vi "Message_Handler.vi"(7 "Action":T5, 8 "error in (no error)":errorcluster, 9 "Time_Out":i32, 11 "Message_IN":T1) -> (0 "error out":errorcluster, 3 "Message_OUT":T1)   [LabVIEW 2024, in "Camera.lvlib" / "Message_Handler.lvlib"]
uses:
  Message_Handler.lvlib
  typedeff_CommunicationModuleAction.ctl
  typedeff_Message.ctl
  typedeff_Message_Command.ctl
  typedeff_Message_Parameters.ctl
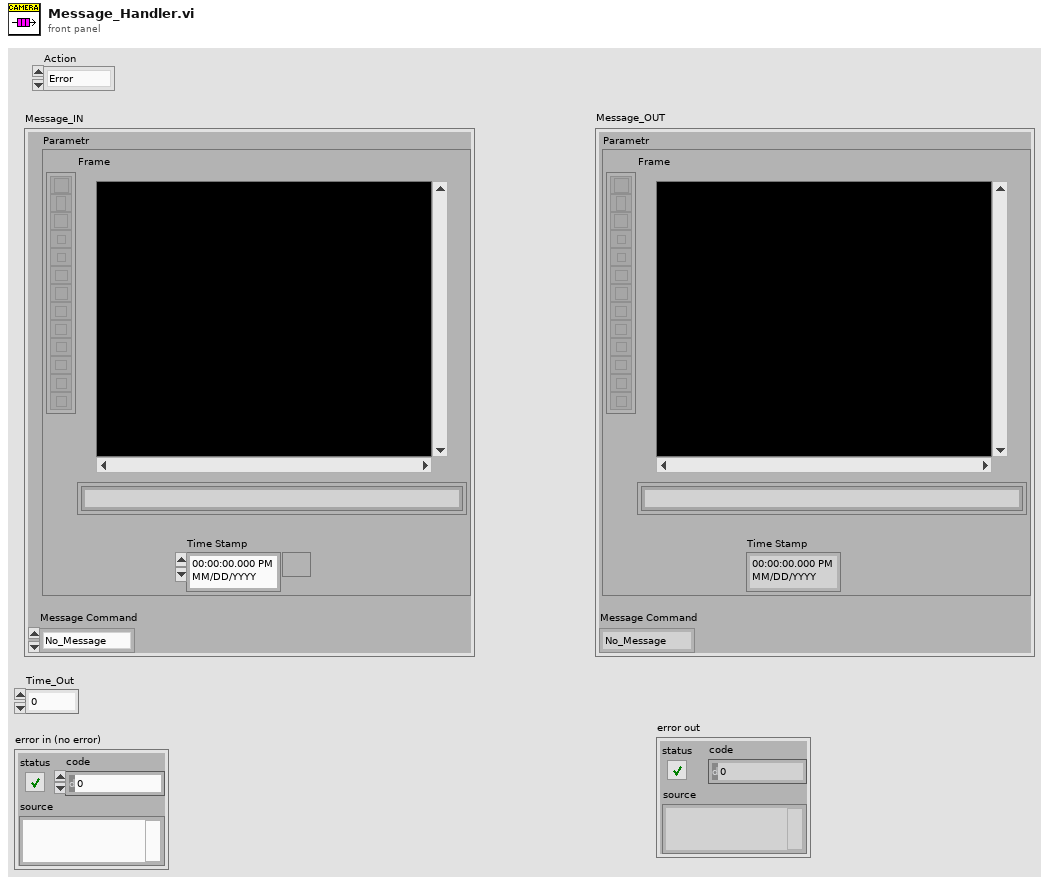
[diagram p1: front panel]
types:
  T1 = typedef "Camera.lvlib/Message_Handler.lvlib/typedeff_Message.ctl" = cluster{"Message Command":T2, "Parametr":T3}
  T2 = typedef "Camera.lvlib/Message_Handler.lvlib/typedeff_Message_Command.ctl" = enum16{"No_Message", "Send_photo"}
  T3 = typedef "Camera.lvlib/Message_Handler.lvlib/typedeff_Message_Parameters.ctl" = cluster{"Frame":T4, "Time Stamp":timestamp}
  T4 = typedef "IMAQ Image.ctl" = refnum<image>
  T5 = typedef "Camera.lvlib/Message_Handler.lvlib/typedeff_CommunicationModuleAction.ctl" = enum16{"Error", "Init", "Send Msg", "Recive Msg", "Shut Down"}
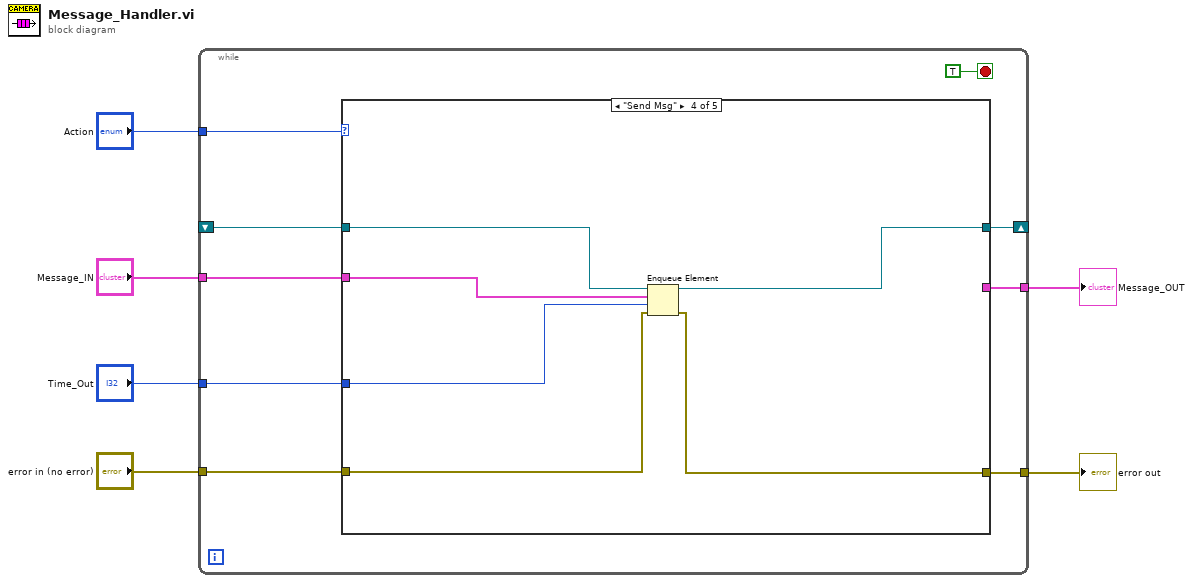
[diagram p0: block diagram]
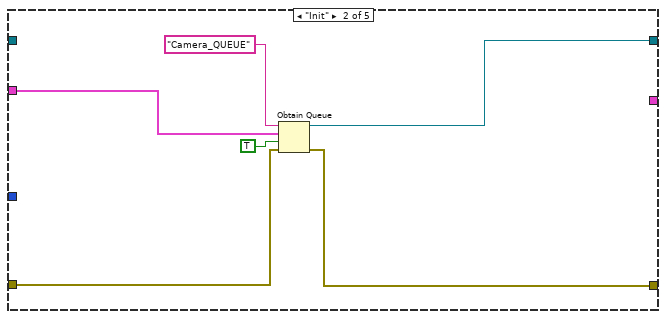
[diagram p3: hidden frame]
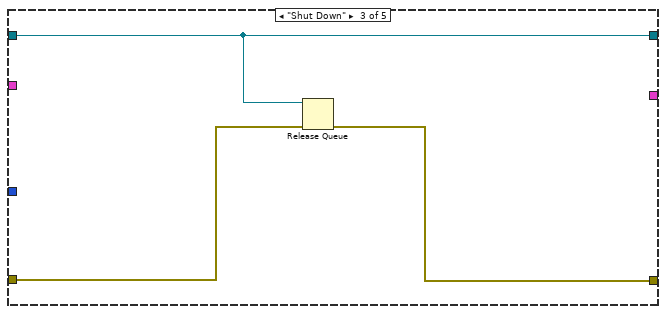
[diagram p4: hidden frame]
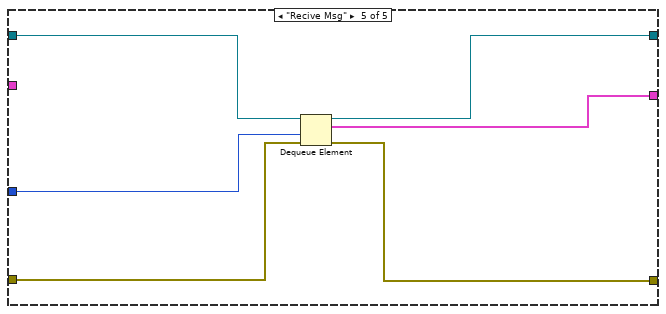
[diagram p5: hidden frame]
diagram:
  n1 = while {
    tunnel: "Action" -> [w14]
    tunnel: "error in (no error)" -> [w13]
    shift-right: [w12] -> _
    shift-left: _ -> [w11]
    tunnel: [w10] -> w4
    tunnel: "Time_Out" -> [w9]
    tunnel: [w8] -> w2
    tunnel: "Message_IN" -> [w7]
    stop <- TRUE stop-if-true
    n2 = case shown="\"Send Msg\"" w14 {
      tunnel: w13 -> [_ w21 w25 w28 w32]
      tunnel: [w16 w20 w23 w29 w35] -> w12
      tunnel: w11 -> [w16 _ w23 w31 w37]
      tunnel: [_ w19 w24 w27 w33] -> w10
      tunnel: w9 -> [_ _ _ w30 w36]
      tunnel: [_ _ _ _ w34] -> w8
      tunnel: w7 -> [_ w17 _ w26 _]
      frame "Error", Default {
      }
      frame "Init" {
        n3 = Obtain Queue(name (unnamed)="Camera_QUEUE", element data type=w17, create if not found? (T)=TRUE, error in (no error)=w21) -> (queue out=w20:refnum<queue>, error out=w19:errorcluster)  [unwired: 1 in, 1 out]
      }
      frame "Shut Down" {
        n4 = Release Queue(queue=w23, error in (no error)=w25) -> (error out=w24:errorcluster)  [unwired: 1 in, 2 out]
      }
      frame "Send Msg" {
        n5 = Enqueue Element(queue=w31, element=w26, timeout in ms (-1)=w30, error in (no error)=w28) -> (queue out=w29:refnum<queue>, error out=w27:errorcluster)  [unwired: 1 out]
      }
      frame "Recive Msg" {
        n6 = Dequeue Element(queue=w37, timeout in ms (-1)=w36, error in (no error)=w32) -> (queue out=w35:refnum<queue>, element=w34:T1, error out=w33:errorcluster)  [unwired: 1 out]
      }
    }
  }
  "error out" <- w4
  "Message_OUT" <- w2
